vi "GraphSettings_stm.vi"(8 "error in":errorcluster, 9 "StateMachineSteps":T1[](array[typedef]) {"STM Graph"."Lines"."Color" format="%x"}, 10 "FNs":enum16{"Back", "Front", "Replace"}(ring), 11 "queue in":refnum<queue>) -> (0 "error out":errorcluster, 3 "queue out":refnum<queue>)   [LabVIEW 2018]
uses:
  GraphSettings_STM.ctl
  GraphSettings_ITEM.ctl
  CTL/STM GRAPH.ctl
  CTL/Graph settings.ctl
  CTL/Line.ctl
  View.ctl
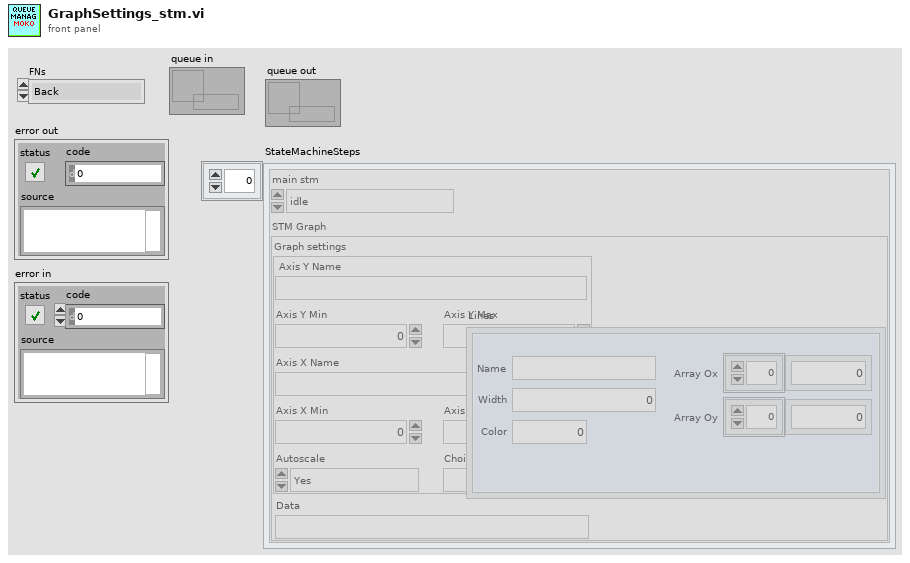
[diagram p1: front panel]
types:
  T1 = typedef "GraphSettings_STM.ctl" = cluster{"main stm":T2, "STM Graph":T3}
  T2 = typedef "GraphSettings_ITEM.ctl" = enum16{"idle", "init", "close", "_____ SETTINGS _____ ", "Receive Data", "Send Data", "Change Line", "Delete Line", "Add Line", "FrontPanelWindowState", "Change Color", "Choice Line"}
  T3 = typedef "STM GRAPH.ctl" = cluster{"Graph settings":T4, "Lines":T5[], "Data":string}
  T4 = typedef "Graph settings.ctl" = cluster{"Axis X Min":dbl, "Axis X Name":string, "Axis X Max":dbl, "Axis Y Min":dbl, " Axis Y Name":string, "Axis Y Max":dbl, "Autoscale":enum16{"Yes", "No", "Only Oy", "Only Ox"}, "Choice Line":dbl}
  T5 = typedef "Line.ctl" = cluster{"Width":dbl, "Color":i64, "Array Oy":dbl[], "Array Ox":dbl[], "Name":string, "Plot Visible":T6}
  T6 = typedef "View.ctl" = bool
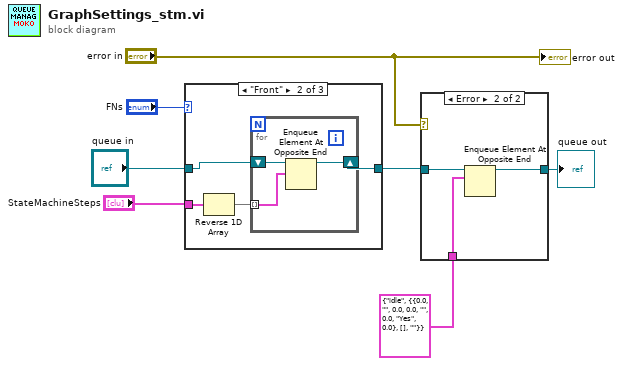
[diagram p0: block diagram]
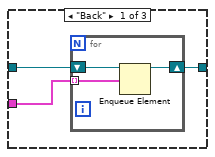
[diagram p3: hidden frame]
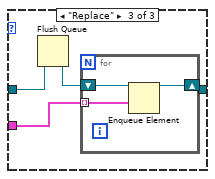
[diagram p4: hidden frame]
diagram:
  n1 = case shown="\"Front\"" "FNs" {
    tunnel: "StateMachineSteps" -> [w9 w15 w23]
    tunnel: [w10 w16 w22] -> w6
    tunnel: "queue in" -> [w8 w14 w21]
    frame "Back" {
      n2 = for {
        shift-right: [w13] -> w10
        shift-left: w8 -> [w11]
        tunnel: w9 -> [w12] mode=indexing
        n3 = Enqueue Element(queue=w11, element=w12) -> (queue out=w13:refnum<queue>)  [unwired: 2 in, 2 out]
      }
    }
    frame "Front" {
      n4 = Reverse 1D Array(array=w15) -> (reversed array=w17:T1[])
      n5 = for {
        tunnel: w17 -> [w19] mode=indexing
        shift-right: [w18] -> w16
        shift-left: w14 -> [w20]
        n6 = Enqueue Element At Opposite End(queue=w20, element=w19) -> (queue out=w18:refnum<queue>)  [unwired: 2 in, 2 out]
      }
    }
    frame "Replace" {
      n7 = Flush Queue(queue=w21) -> (queue out=w24:refnum<queue>)  [unwired: 1 in, 2 out]
      n8 = for {
        tunnel: w23 -> [w26] mode=indexing
        shift-right: [w25] -> w22
        shift-left: w24 -> [w27]
        n9 = Enqueue Element(queue=w27, element=w26) -> (queue out=w25:refnum<queue>)  [unwired: 2 in, 2 out]
      }
    }
  }
  n10 = case shown="Error" "error in" {
    tunnel: w6 -> [w28 w31]
    tunnel: [w28 w30] -> w1
    tunnel: T1 {"main stm"=enum."idle", "STM Graph"={"Graph settings"={"Axis X Min"=0.0, "Axis X Name"="", "Axis X Max"=0.0, "Axis Y Min"=0.0, " Axis Y Name"="", "Axis Y Max"=0.0, "Autoscale"=enum."Yes", "Choice Line"=0.0}, "Lines"=[], "Data"=""}} ("element") -> [_ w29]
    frame No Error {
    }
    frame Error {
      n11 = Enqueue Element At Opposite End(queue=w31, element=w29) -> (queue out=w30:refnum<queue>)  [unwired: 2 in, 2 out]
    }
  }
  "queue out" <- w1
  "error out" <- "error in"
